vi "log analysis_gps.vi"() -> ()   [LabVIEW 2019] (continued)
0.4317,0.3028,0.5934,0.1135,0.0949,0.0816,0.0957,0.0998,5.2642,0f000001,0*80882a82\n\t", "INSPVAXA,USB3,0,48.5,FINESTEERING,2107,283990.000,02000000,471d,15824;INS_ALIGNMENT_COMPLETE,INS_RTKFIXED,37.37029204407,126.72099699457,9.6988,22.3000,-0.3771,-0.2894,0.0402,-1.247584491,0.667932801,212.987583360,0.4317,0.3028,0.5934,0.1135,0.0949,0.0816,0.0957,0.0998,5.2642,0f000001,0*cfed9a10\n\t", "INSPVAXA,USB3,0,50.0,FINESTEERING,2107,283990.500,02000000,471d,15824;INS_ALIGNMENT_COMPLETE,INS_RTKFIXED,37.37029029580,126.72099542809,9.7025,22.3000,-0.3670,-0.2925,0.0054,-1.144620935,0.833749283,212.845661627,0.4315,0.3031,0.5931,0.1131,0.0946,0.0813,0.0957,0.0998,5.2654,0f000001,0*19c2a41b\n\t", "INSPVAXA,USB3,0,50.0,FINESTEERING,2107,283991.000,02000000,471d,15824;INS_ALIGNMENT_COMPLETE,INS_RTKFIXED,37.37028854245,126.72099383471,9.7082,22.3000,-0.3734,-0.2981,0.0505,-1.053794581,0.860705414,212.916628462,0.4315,0.3031,0.5931,0.1131,0.0946,0.0813,0.0957,0.0998,5.2654,0f000001,0*6cd9c21a\n\t", "INSPVAXA,USB3,0,50.0,FINESTEERING,2107,283991.500,02000000,471d,15824;INS_ALIGNMENT_COMPLETE,INS_RTKFIXED,37.37028678118,126.72099223881,9.7128,22.3000,-0.3905,-0.2870,0.0338,-1.308863276,0.828346639,212.947096436,0.4317,0.3031,0.5932,0.1128,0.0940,0.0810,0.0956,0.0998,5.2662,0f000001,0*9682182f\n\t", "INSPVAXA,USB3,0,50.0,FINESTEERING,2107,283992.000,02000000,471d,15824;INS_ALIGNMENT_COMPLETE,INS_RTKFIXED,37.37028506885,126.72099063831,9.7202,22.3000,-0.3587,-0.3008,0.0194,-1.224018986,0.834141555,212.863695719,0.4317,0.3031,0.5932,0.1128,0.0940,0.0810,0.0956,0.0998,5.2662,0f000001,0*43bde827\n\t", "INSPVAXA,USB3,0,45.0,FINESTEERING,2107,283992.500,02000000,471d,15824;INS_ALIGNMENT_COMPLETE,INS_RTKFIXED,37.37028333459,126.72098904452,9.7257,22.3000,-0.3784,-0.2965,0.0443,-1.050562507,0.745679158,212.979675556,0.4319,0.3033,0.5933,0.1130,0.0942,0.0816,0.0956,0.0997,5.2672,0f000001,0*f6d38c7c\n\t", "INSPVAXA,USB3,0,45.0,FINESTEERING,2107,283993.000,02000000,471d,15824;INS_ALIGNMENT_COMPLETE,INS_RTKFIXED,37.37028161694,126.72098748507,9.7305,22.3000,-0.3588,-0.2835,0.0413,-1.341951739,0.883295300,213.030480888,0.4319,0.3033,0.5933,0.1130,0.0942,0.0816,0.0956,0.0997,5.2672,0f000001,0*8bfaad14\n\t", "INSPVAXA,USB3,0,49.0,FINESTEERING,2107,283993.500,02000000,471d,15824;INS_ALIGNMENT_COMPLETE,INS_RTKFIXED,37.37027987729,126.72098589860,9.7339,22.3000,-0.3886,-0.3118,0.0118,-1.186705860,0.635599144,213.040521206,0.4318,0.3035,0.5934,0.1127,0.0938,0.0813,0.0956,0.0997,5.2685,0f000001,0*5b9abbf8\n\t", "INSPVAXA,USB3,0,49.0,FINESTEERING,2107,283994.000,02000000,471d,15824;INS_ALIGNMENT_COMPLETE,INS_RTKFIXED,37.37027813856,126.72098430051,9.7386,22.3000,-0.3794,-0.2983,0.0413,-1.126640911,0.427805755,213.093758144,0.4318,0.3035,0.5934,0.1127,0.0938,0.0813,0.0956,0.0997,5.2685,0f000001,0*e42dd86e\n\t", "INSPVAXA,USB3,0,41.5,FINESTEERING,2107,283994.500,02000000,471d,15824;INS_ALIGNMENT_COMPLETE,INS_RTKFIXED,37.37027639241,126.72098271837,9.7433,22.3000,-0.3724,-0.2941,0.0395,-1.023992417,0.392331965,213.143460080,0.4318,0.3036,0.5935,0.1130,0.0944,0.0820,0.0956,0.0997,5.2698,0f000001,0*0337d50d\n\t", "INSPVAXA,USB3,0,41.5,FINESTEERING,2107,283995.000,02000000,471d,15824;INS_ALIGNMENT_COMPLETE,INS_RTKFIXED,37.37027465637,126.72098113948,9.7472,22.3000,-0.3708,-0.2998,0.0087,-1.064940932,0.419900141,213.213279076,0.4318,0.3036,0.5935,0.1130,0.0944,0.0820,0.0956,0.0997,5.2698,0f000001,0*335ddb23\n\t", "INSPVAXA,USB3,0,49.5,FINESTEERING,2107,283995.500,02000000,471d,15824;INS_ALIGNMENT_COMPLETE,INS_RTKFIXED,37.37027293232,126.72097957470,9.7494,22.3000,-0.3727,-0.2928,0.0273,-1.114629129,0.419021826,213.334562050,0.4319,0.3032,0.5939,0.1127,0.0939,0.0817,0.0957,0.0997,5.2708,0f000001,0*bec96f91\n\t", "INSPVAXA,USB3,0,49.5,FINESTEERING,2107,283996.000,02000000,471d,15824;INS_ALIGNMENT_COMPLETE,INS_RTKFIXED,37.37027121924,126.72097799640,9.7538,22.3000,-0.3785,-0.2972,0.0344,-0.912805448,0.531088142,213.375963340,0.4319,0.3032,0.5939,0.1127,0.0939,0.0817,0.0957,0.0997,5.2708,0f000001,0*e0fc992c\n\t", "INSPVAXA,USB3,0,48.5,FINESTEERING,2107,283996.500,02000000,471d,15824;INS_ALIGNMENT_COMPLETE,INS_RTKFIXED,37.37026950707,126.72097642523,9.7575,22.3000,-0.3790,-0.2971,0.0045,-1.031000712,0.442701672,213.487798192,0.4317,0.3031,0.5940,0.1124,0.0936,0.0813,0.0957,0.0997,5.2719,0f000001,0*6ebbd163\n\t", "INSPVAXA,USB3,0,48.5,FINESTEERING,2107,283997.000,02000000,471d,15824;INS_ALIGNMENT_COMPLETE,INS_RTKFIXED,37.37026778904,126.72097482944,9.7613,22.3000,-0.3776,-0.3087,0.0370,-1.077110117,0.533414002,213.644467670,0.4317,0.3031,0.5940,0.1124,0.0936,0.0813,0.0957,0.0997,5.2719,0f000001,0*eda6f981\n\t", "INSPVAXA,USB3,0,51.5,FINESTEERING,2107,283997.500,02000000,471d,15824;INS_ALIGNMENT_COMPLETE,INS_RTKFIXED,37.37026610502,126.72097322741,9.7652,22.3000,-0.3735,-0.2926,0.0418,-0.879042002,0.635388403,213.712940335,0.4318,0.3033,0.5943,0.1122,0.0934,0.0810,0.0958,0.0998,5.2733,0f000001,0*c5914784\n\t", "INSPVAXA,USB3,0,51.5,FINESTEERING,2107,283998.000,02000000,471d,15824;INS_ALIGNMENT_COMPLETE,INS_RTKFIXED,37.37026439172,126.72097159305,9.7705,22.3000,-0.3793,-0.3043,0.0231,-0.804340415,0.481108177,213.810502820,0.4318,0.3033,0.5943,0.1122,0.0934,0.0810,0.0958,0.0998,5.2733,0f000001,0*97086bfc\n\t", "INSPVAXA,USB3,0,51.0,FINESTEERING,2107,283998.500,02000000,471d,15824;INS_ALIGNMENT_COMPLETE,INS_RTKFIXED,37.37026268780,126.72097001383,9.7729,22.3000,-0.3715,-0.3065,0.0247,-0.969252583,0.581649669,213.913706075,0.4317,0.3034,0.5943,0.1125,0.0938,0.0813,0.0958,0.0998,5.2748,0f000001,0*e268e54b\n\t", "INSPVAXA,USB3,0,51.0,FINESTEERING,2107,283999.000,02000000,471d,15824;INS_ALIGNMENT_COMPLETE,INS_RTKFIXED,37.37026095503,126.72096836486,9.7766,22.3000,-0.3661,-0.3031,0.0412,-0.630265217,0.537624421,214.046710084,0.4317,0.3034,0.5943,0.1125,0.0938,0.0813,0.0958,0.0998,5.2748,0f000001,0*95a9afe3\n\t", "INSPVAXA,USB3,0,49.5,FINESTEERING,2107,283999.500,02000000,471d,15824;INS_ALIGNMENT_COMPLETE,INS_RTKFIXED,37.37025925101,126.72096675133,9.7788,22.3000,-0.3833,-0.2925,0.0276,-0.676998170,0.665326171,214.262149706,0.4315,0.3034,0.5944,0.1124,0.0937,0.0810,0.0958,0.0998,5.2762,0f000001,0*6af82f9f\n\t", "DUALANTENNAHEADINGA,USB3,0,49.5,FINESTEERING,2107,284000.000,02000000,d426,15824;INSUFFICIENT_OBS,NONE,-1.000000000,0.000000000,0.000000000,0.0,0.000000000,0.000000000,\"631T\",10,3,3,3,04,00,20,00*77bc98b4\n\t", "INSPVAXA,USB3,0,51.5,FINESTEERING,2107,284000.500,02000000,471d,15824;INS_ALIGNMENT_COMPLETE,INS_RTKFIXED,37.37025584789,126.72096350983,9.7893,22.3000,-0.3628,-0.2938,0.0413,-0.857969709,0.678060682,214.382554495,0.4312,0.3037,0.5943,0.1122,0.0935,0.0807,0.0958,0.0998,5.2776,0f000001,0*ebd8e3c0\n\t", "INSPVAXA,USB3,0,51.5,FINESTEERING,2107,284001.000,02000000,471d,15824;INS_ALIGNMENT_COMPLETE,INS_RTKFIXED,37.37025415125,126.72096186926,9.7945,22.3000,-0.3741,-0.3078,0.0321,-0.868538574,0.838914865,214.492970647,0.4312,0.3037,0.5943,0.1122,0.0935,0.0807,0.0958,0.0998,5.2776,0f000001,0*3e03e893\n\t", "INSPVAXA,USB3,0,51.5,FINESTEERING,2107,284001.500,02000000,471d,15824;INS_ALIGNMENT_COMPLETE,INS_RTKFIXED,37.37025245958,126.72096024152,9.7991,22.3000,-0.3759,-0.3085,0.0182,-0.727729305,0.679989814,214.645667926,0.4313,0.3035,0.5942,0.1121,0.0935,0.0804,0.0958,0.0999,5.2791,0f000001,0*dc1168a6\n\t", "INSPVAXA,USB3,0,51.5,FINESTEERING,2107,284002.000,02000000,471d,15824;INS_ALIGNMENT_COMPLETE,INS_RTKFIXED,37.37025076480,126.72095861170,9.8045,22.3000,-0.3744,-0.3095,0.0470,-0.816843186,0.787318201,214.620444446,0.4313,0.3035,0.5942,0.1121,0.0935,0.0804,0.0958,0.0999,5.2791,0f000001,0*a2e8b743\n\t", "INSPVAXA,USB3,0,51.5,FINESTEERING,2107,284002.500,02000000,471d,15824;INS_ALIGNMENT_COMPLETE,INS_RTKFIXED,37.37024907128,126.72095697824,9.8087,22.3000,-0.3691,-0.2994,0.0299,-0.885724025,0.937533929,214.679042241,0.4311,0.3036,0.5939,0.1121,0.0934,0.0802,0.0958,0.0999,5.2806,0f000001,0*c448775c\n\t", "INSPVAXA,USB3,0,51.5,FINESTEERING,2107,284003.000,02000000,471d,15824;INS_ALIGNMENT_COMPLETE,INS_RTKFIXED,37.37024737149,126.72095529976,9.8122,22.3000,-0.3776,-0.3159,0.0244,-0.547028991,0.805451972,214.632048591,0.4311,0.3036,0.5939,0.1121,0.0934,0.0802,0.0958,0.0999,5.2806,0f000001,0*63822f21\n\t", "INSPVAXA,USB3,0,51.5,FINESTEERING,2107,284003.500,02000000,471d,15824;INS_ALIGNMENT_COMPLETE,INS_RTKFIXED,37.37024569352,126.72095368049,9.8164,22.3000,-0.3735,-0.3059,0.0298,-0.766116345,0.775309427,214.637421132,0.4311,0.3038,0.5936,0.1120,0.0934,0.0800,0.0957,0.0999,5.2822,0f000001,0*13581e5f\n\t", "INSPVAXA,USB3,0,51.5,FINESTEERING,2107,284004.000,02000000,471d,15824;INS_ALIGNMENT_COMPLETE,INS_RTKFIXED,37.37024397579,126.72095202035,9.8197,22.3000,-0.3785,-0.3116,0.0275,-0.938815319,0.810465745,214.701472535,0.4311,0.3038,0.5936,0.1120,0.0934,0.0800,0.0957,0.0999,5.2822,0f000001,0*789baddb\n\t", "DUALANTENNAHEADINGA,USB3,0,47.5,FINESTEERING,2107,284004.500,02000000,d426,15824;INSUFFICIENT_OBS,NONE,-1.000000000,0.000000000,0.000000000,0.0,0.000000000,0.000000000,\"631T\",10,3,3,3,04,00,20,00*da91d4f3\n\t", "INSPVAXA,USB3,0,47.5,FINESTEERING,2107,284005.000,02000000,471d,15824;INS_ALIGNMENT_COMPLETE,INS_RTKFIXED,37.37024061401,126.72094879160,9.8273,22.3000,-0.3519,-0.2880,0.0226,-1.106323237,0.920552674,214.656768250,0.4310,0.3041,0.5933,0.1128,0.0943,0.0811,0.0957,0.0998,5.2837,0f000001,0*6ae8f33a\n\t", "DUALANTENNAHEADINGA,USB3,0,51.5,FINESTEERING,2107,284005.500,02000000,d426,15824;INSUFFICIENT_OBS,NONE,-1.000000000,0.000000000,0.000000000,0.0,0.000000000,0.000000000,\"631T\",10,3,3,3,04,00,20,00*e47d0294\n\t", "DUALANTENNAHEADINGA,USB3,0,51.5,FINESTEERING,2107,284006.000,02000000,d426,15824;INSUFFICIENT_OBS,NONE,-1.000000000,0.000000000,0.000000000,0.0,0.000000000,0.000000000,\"631T\",11,3,3,3,04,00,20,00*52e49efe\n\t", "INSPVAXA,USB3,0,53.0,FINESTEERING,2107,284006.500,02000000,471d,15824;INS_ALIGNMENT_COMPLETE,INS_RTKFIXED,37.37023555537,126.72094390060,9.8375,22.3000,-0.3979,-0.3155,0.0300,-1.049604395,0.780641756,214.313549456,0.4317,0.3045,0.5932,0.1125,0.0938,0.0806,0.0956,0.0998,5.2867,0f000001,0*baf56160\n\t", "DUALANTENNAHEADINGA,USB3,0,53.0,FINESTEERING,2107,284007.000,02000000,d426,15824;INSUFFICIENT_OBS,NONE,-1.000000000,0.000000000,0.000000000,0.0,0.000000000,0.000000000,\"631T\",11,3,3,3,04,00,20,00*a2cfd1a3\n\t", "INSPVAXA,USB3,0,51.5,FINESTEERING,2107,284007.500,02000000,471d,15824;INS_ALIGNMENT_COMPLETE,INS_RTKFIXED,37.37023216601,126.72094065037,9.8419,22.3000,-0.3656,-0.2859,0.0240,-0.929585052,0.783187506,214.018400547,0.4319,0.3042,0.5932,0.1130,0.0943,0.0814,0.0956,0.0998,5.2881,0f000001,0*b155cbfb\n\t", "INSPVAXA,USB3,0,51.5,FINESTEERING,2107,284008.000,02000000,471d,15824;INS_ALIGNMENT_COMPLETE,INS_RTKFIXED,37.37023049066,126.72093905511,9.8436,22.3000,-0.3675,-0.2972,0.0326,-1.081497544,1.069523498,213.947516981,0.4319,0.3042,0.5932,0.1130,0.0943,0.0814,0.0956,0.0998,5.2881,0f000001,0*b15b7ce2\n\t", "DUALANTENNAHEADINGA,USB3,0,50.5,FINESTEERING,2107,284008.500,02000000,d426,15824;INSUFFICIENT_OBS,NONE,-1.000000000,0.000000000,0.000000000,0.0,0.000000000,0.000000000,\"631T\",10,3,3,3,04,00,20,00*59d2ef86\n\t", "INSPVAXA,USB3,0,50.5,FINESTEERING,2107,284009.000,02000000,471d,15824;INS_ALIGNMENT_COMPLETE,INS_RTKFIXED,37.37022706155,126.72093581324,9.8448,22.3000,-0.3775,-0.3022,0.0342,-1.257860345,0.478173626,213.753744794,0.4320,0.3040,0.5934,0.1130,0.0939,0.0812,0.0956,0.0998,5.2894,0f000001,0*088bd23f\n\t", "DUALANTENNAHEADINGA,USB3,0,50.0,FINESTEERING,2107,284009.500,02000000,d426,15824;INSUFFICIENT_OBS,NONE,-1.000000000,0.000000000,0.000000000,0.0,0.000000000,0.000000000,\"631T\",12,3,3,3,04,00,20,00*15c40b62\n\t", "DUALANTENNAHEADINGA,USB3,0,50.0,FINESTEERING,2107,284010.000,02000000,d426,15824;INSUFFICIENT_OBS,NONE,-1.000000000,0.000000000,0.000000000,0.0,0.000000000,0.000000000,\"631T\",11,3,3,3,04,00,20,00*2b190075\n\t", "DUALANTENNAHEADINGA,USB3,0,52.0,FINESTEERING,2107,284010.500,02000000,d426,15824;INSUFFICIENT_OBS,NONE,-1.000000000,0.000000000,0.000000000,0.0,0.000000000,0.000000000,\"631T\",11,3,3,3,04,00,20,00*3483bc64\n\t", "DUALANTENNAHEADINGA,USB3,0,52.0,FINESTEERING,2107,284011.000,02000000,d426,15824;INSUFFICIENT_OBS,NONE,-1.000000000,0.000000000,0.000000000,0.0,0.000000000,0.000000000,\"631T\",10,3,3,3,04,00,20,00*59aa29bc\n\t", "DUALANTENNAHEADINGA,USB3,0,50.0,FINESTEERING,2107,284011.500,02000000,d426,15824;INSUFFICIENT_OBS,NONE,-1.000000000,0.000000000,0.000000000,0.0,0.000000000,0.000000000,\"631T\",10,3,3,3,04,00,20,00*463095ad\n\t", "DUALANTENNAHEADINGA,USB3,0,50.0,FINESTEERING,2107,284012.000,02000000,d426,15824;INSUFFICIENT_OBS,NONE,-1.000000000,0.000000000,0.000000000,0.0,0.000000000,0.000000000,\"631T\",11,3,3,3,04,00,20,00*f0a909c7\n\t", "INSPVAXA,USB3,0,52.0,FINESTEERING,2107,284012.500,02000000,471d,15824;INS_ALIGNMENT_COMPLETE,INS_RTKFIXED,37.37021521893,126.72092466142,9.8618,22.3000,-0.3847,-0.3021,0.0234,-0.775837810,0.832251652,213.741589159,0.4316,0.3037,0.5939,0.1121,0.0935,0.0807,0.0957,0.0997,5.2927,0f000001,0*15662a94\n\t", "DUALANTENNAHEADINGA,USB3,0,52.0,FINESTEERING,2107,284013.000,02000000,d426,15824;INSUFFICIENT_OBS,NONE,-1.000000000,0.000000000,0.000000000,0.0,0.000000000,0.000000000,\"631T\",11,3,3,3,04,00,20,00*55f8a056\n\t", "DUALANTENNAHEADINGA,USB3,0,49.0,FINESTEERING,2107,284013.500,02000000,d426,15824;INSUFFICIENT_OBS,NONE,-1.000000000,0.000000000,0.000000000,0.0,0.000000000,0.000000000,\"631T\",10,3,3,3,04,00,20,00*bcdfd03e\n\t", "DUALANTENNAHEADINGA,USB3,0,49.0,FINESTEERING,2107,284014.000,02000000,d426,15824;INSUFFICIENT_OBS,NONE,-1.000000000,0.000000000,0.000000000,0.0,0.000000000,0.000000000,\"631T\",10,3,3,3,04,00,20,00*b1b5d929\n\t", "DUALANTENNAHEADINGA,USB3,0,48.0,FINESTEERING,2107,284014.500,02000000,d426,15824;INSUFFICIENT_OBS,NONE,-1.000000000,0.000000000,0.000000000,0.0,0.000000000,0.000000000,\"631T\",11,3,3,3,04,00,20,00*d5009e8c\n\t", "INSPVAXA,USB3,0,48.0,FINESTEERING,2107,284015.000,02000000,471d,15824;INS_ALIGNMENT_COMPLETE,INS_RTKFIXED,37.37020683430,126.72091660839,9.8841,22.3000,-0.3478,-0.2798,0.0325,-1.211016237,0.525489122,214.520046866,0.4313,0.3041,0.5940,0.1119,0.0933,0.0802,0.0957,0.0997,5.2955,0f000001,0*ac9f229d\n\t", "INSPVAXA,USB3,0,50.5,FINESTEERING,2107,284015.500,02000000,471d,15824;INS_ALIGNMENT_COMPLETE,INS_RTKFIXED,37.37020518291,126.72091499411,9.8875,22.3000,-0.3472,-0.2997,0.0277,-1.071436018,0.954919930,214.713975272,0.4312,0.3037,0.5941,0.1119,0.0933,0.0800,0.0957,0.0997,5.2971,0f000001,0*82bfde41\n\t", "INSPVAXA,USB3,0,50.5,FINESTEERING,2107,284016.000,02000000,471d,15824;INS_ALIGNMENT_COMPLETE,INS_RTKFIXED,37.37020352454,126.72091333889,9.8896,22.3000,-0.3642,-0.3113,0.0147,-0.944083303,0.844230452,215.071518379,0.4312,0.3037,0.5941,0.1119,0.0933,0.0800,0.0957,0.0997,5.2971,0f000001,0*acd4ef81\n\t", "DUALANTENNAHEADINGA,USB3,0,48.0,FINESTEERING,2107,284016.500,02000000,d426,15824;INSUFFICIENT_OBS,NONE,-1.000000000,0.000000000,0.000000000,0.0,0.000000000,0.000000000,\"631T\",11,3,3,3,04,00,20,00*0eb0973e\n\t", "DUALANTENNAHEADINGA,USB3,0,48.0,FINESTEERING,2107,284017.000,02000000,d426,15824;INSUFFICIENT_OBS,NONE,-1.000000000,0.000000000,0.000000000,0.0,0.000000000,0.000000000,\"631T\",10,3,3,3,04,00,20,00*639902e6\n\t", "DUALANTENNAHEADINGA,USB3,0,46.5,FINESTEERING,2107,284017.500,02000000,d426,15824;INSUFFICIENT_OBS,NONE,-1.000000000,0.000000000,0.000000000,0.0,0.000000000,0.000000000,\"631T\",10,3,3,3,04,00,20,00*f7dfbd48\n\t", "DUALANTENNAHEADINGA,USB3,0,46.5,FINESTEERING,2107,284018.000,02000000,d426,15824;INSUFFICIENT_OBS,NONE,-1.000000000,0.000000000,0.000000000,0.0,0.000000000,0.000000000,\"631T\",10,3,3,3,04,00,20,00*22979e15\n\t", "DUALANTENNAHEADINGA,USB3,0,48.0,FINESTEERING,2107,284018.500,02000000,d426,15824;INSUFFICIENT_OBS,NONE,-1.000000000,0.000000000,0.000000000,0.0,0.000000000,0.000000000,\"631T\",11,3,3,3,04,00,20,00*6133a1e3\n\t", "DUALANTENNAHEADINGA,USB3,0,48.0,FINESTEERING,2107,284019.000,02000000,d426,15824;INSUFFICIENT_OBS,NONE,-1.000000000,0.000000000,0.000000000,0.0,0.000000000,0.000000000,\"631T\",13,3,3,3,04,00,20,00*af4cb292\n\t", "DUALANTENNAHEADINGA,USB3,0,50.0,FINESTEERING,2107,284019.500,02000000,d426,15824;INSUFFICIENT_OBS,NONE,-1.000000000,0.000000000,0.000000000,0.0,0.000000000,0.000000000,\"631T\",12,3,3,3,04,00,20,00*eaa6b916\n\t", "DUALANTENNAHEADINGA,USB3,0,50.0,FINESTEERING,2107,284020.000,02000000,d426,15824;INSUFFICIENT_OBS,NONE,-1.000000000,0.000000000,0.000000000,0.0,0.000000000,0.000000000,\"631T\",10,3,3,3,04,00,20,00*262d50f0\n\t", "DUALANTENNAHEADINGA,USB3,0,48.5,FINESTEERING,2107,284020.500,02000000,d426,15824;INSUFFICIENT_OBS,NONE,-1.000000000,0.000000000,0.000000000,0.0,0.000000000,0.000000000,\"631T\",9,3,3,3,04,00,20,00*7dfaf070\n\t", "DUALANTENNAHEADINGA,USB3,0,48.5,FINESTEERING,2107,284021.000,02000000,d426,15824;INSUFFICIENT_OBS,NONE,-1.000000000,0.000000000,0.000000000,0.0,0.000000000,0.000000000,\"631T\",9,3,3,3,04,00,20,00*66d97584\n\t", "DUALANTENNAHEADINGA,USB3,0,51.5,FINESTEERING,2107,284021.500,02000000,d426,15824;INSUFFICIENT_OBS,NONE,-1.000000000,0.000000000,0.000000000,0.0,0.000000000,0.000000000,\"631T\",10,3,3,3,04,00,20,00*add87518\n\t", "DUALANTENNAHEADINGA,USB3,0,51.5,FINESTEERING,2107,284022.000,02000000,d426,15824;INSUFFICIENT_OBS,NONE,-1.000000000,0.000000000,0.000000000,0.0,0.000000000,0.000000000,\"631T\",11,3,3,3,04,00,20,00*1b41e972\n\t", "DUALANTENNAHEADINGA,USB3,0,51.0,FINESTEERING,2107,284022.500,02000000,d426,15824;INSUFFICIENT_OBS,NONE,-1.000000000,0.000000000,0.000000000,0.0,0.000000000,0.000000000,\"631T\",11,3,3,3,04,00,20,00*99281ee7\n\t", "DUALANTENNAHEADINGA,USB3,0,51.0,FINESTEERING,2107,284023.000,02000000,d426,15824;INSUFFICIENT_OBS,NONE,-1.000000000,0.000000000,0.000000000,0.0,0.000000000,0.000000000,\"631T\",11,3,3,3,04,00,20,00*23e30b67\n\t", "DUALANTENNAHEADINGA,USB3,0,48.5,FINESTEERING,2107,284023.500,02000000,d426,15824;INSUFFICIENT_OBS,NONE,-1.000000000,0.000000000,0.000000000,0.0,0.000000000,0.000000000,\"631T\",11,3,3,3,04,00,20,00*80d5b0d3\n\t", "DUALANTENNAHEADINGA,USB3,0,50.5,FINESTEERING,2107,284025.000,02000000,d426,15824;INSUFFICIENT_OBS,NONE,-1.000000000,0.000000000,0.000000000,0.0,0.000000000,0.000000000,\"631T\",12,3,3,3,04,00,20,00*062aa131\n\t", "DUALANTENNAHEADINGA,USB3,0,50.0,FINESTEERING,2107,284025.500,02000000,d426,15824;INSUFFICIENT_OBS,NONE,-1.000000000,0.000000000,0.000000000,0.0,0.000000000,0.000000000,\"631T\",11,3,3,3,04,00,20,00*2715d00d\n\t", "DUALANTENNAHEADINGA,USB3,0,50.0,FINESTEERING,2107,284026.000,02000000,d426,15824;INSUFFICIENT_OBS,NONE,-1.000000000,0.000000000,0.000000000,0.0,0.000000000,0.000000000,\"631T\",11,3,3,3,04,00,20,00*466ecc3f\n\t", "DUALANTENNAHEADINGA,USB3,0,52.0,FINESTEERING,2107,284026.500,02000000,d426,15824;INSUFFICIENT_OBS,NONE,-1.000000000,0.000000000,0.000000000,0.0,0.000000000,0.000000000,\"631T\",11,3,3,3,04,00,20,00*59f4702e\n\t", "DUALANTENNAHEADINGA,USB3,0,52.0,FINESTEERING,2107,284027.000,02000000,d426,15824;INSUFFICIENT_OBS,NONE,-1.000000000,0.000000000,0.000000000,0.0,0.000000000,0.000000000,\"631T\",11,3,3,3,04,00,20,00*e33f65ae\n\t", "DUALANTENNAHEADINGA,USB3,0,51.0,FINESTEERING,2107,284027.500,02000000,d426,15824;INSUFFICIENT_OBS,NONE,-1.000000000,0.000000000,0.000000000,0.0,0.000000000,0.000000000,\"631T\",11,3,3,3,04,00,20,00*98e10f1b\n\t", "DUALANTENNAHEADINGA,USB3,0,51.0,FINESTEERING,2107,284028.000,02000000,d426,15824;INSUFFICIENT_OBS,NONE,-1.000000000,0.000000000,0.000000000,0.0,0.000000000,0.000000000,\"631T\",12,3,3,3,04,00,20,00*eeffaaef\n\t", "INSPVAXA,USB3,0,53.0,FINESTEERING,2107,284028.500,02000000,471d,15824;INS_ALIGNMENT_COMPLETE,INS_RTKFIXED,37.37016418129,126.72086876057,9.9277,22.3000,-0.3056,-0.3533,0.0249,-0.407357683,-0.326305353,221.094375999,0.4345,0.3056,0.5971,0.1128,0.0942,0.0822,0.0958,0.1003,5.3097,0f000001,0*9e144474\n\t", "DUALANTENNAHEADINGA,USB3,0,53.0,FINESTEERING,2107,284029.000,02000000,d426,15824;INSUFFICIENT_OBS,NONE,-1.000000000,0.000000000,0.000000000,0.0,0.000000000,0.000000000,\"631T\",11,3,3,3,04,00,20,00*e8f885d7\n\t", "DUALANTENNAHEADINGA,USB3,0,48.5,FINESTEERING,2107,284029.500,02000000,d426,15824;INSUFFICIENT_OBS,NONE,-1.000000000,0.000000000,0.000000000,0.0,0.000000000,0.000000000,\"631T\",11,3,3,3,04,00,20,00*8347932b\n\t", "DUALANTENNAHEADINGA,USB3,0,48.5,FINESTEERING,2107,284030.000,02000000,d426,15824;INSUFFICIENT_OBS,NONE,-1.000000000,0.000000000,0.000000000,0.0,0.000000000,0.000000000,\"631T\",13,3,3,3,04,00,20,00*6a781864\n\t", "DUALANTENNAHEADINGA,USB3,0,50.0,FINESTEERING,2107,284030.500,02000000,d426,15824;INSUFFICIENT_OBS,NONE,-1.000000000,0.000000000,0.000000000,0.0,0.000000000,0.000000000,\"631T\",15,3,3,3,04,00,20,00*30d67e67\n\t", "DUALANTENNAHEADINGA,USB3,0,50.0,FINESTEERING,2107,284031.000,02000000,d426,15824;INSUFFICIENT_OBS,NONE,-1.000000000,0.000000000,0.000000000,0.0,0.000000000,0.000000000,\"631T\",14,3,3,3,04,00,20,00*5dffebbf\n\t", "DUALANTENNAHEADINGA,USB3,0,46.0,FINESTEERING,2107,284031.500,02000000,d426,15824;INSUFFICIENT_OBS,NONE,-1.000000000,0.000000000,0.000000000,0.0,0.000000000,0.000000000,\"631T\",14,3,3,3,04,00,20,00*d9d82858\n\t", "DUALANTENNAHEADINGA,USB3,0,46.0,FINESTEERING,2107,284032.000,02000000,d426,15824;INSUFFICIENT_OBS,NONE,-1.000000000,0.000000000,0.000000000,0.0,0.000000000,0.000000000,\"631T\",15,3,3,3,04,00,20,00*6f41b432\n\t", "INSPVAXA,USB3,0,49.0,FINESTEERING,2107,284032.550,02000000,471d,15824;INS_ALIGNMENT_COMPLETE,INS_RTKFIXED,37.37015203193,126.72085320398,9.9212,22.3000,-0.2929,-0.3693,0.0073,-0.969546435,-0.769890504,222.991083315,0.4327,0.3047,0.5976,0.1132,0.0946,0.0822,0.0960,0.1005,5.3138,0f000001,0*7ab4b638\n\t", "INSPVAXA,USB3,0,49.0,FINESTEERING,2107,284033.050,02000000,471d,15824;INS_ALIGNMENT_COMPLETE,INS_RTKFIXED,37.37015056233,126.72085129060,9.9204,22.3000,-0.2846,-0.3575,0.0263,-1.291425678,-0.544067497,223.276181185,0.4326,0.3039,0.5975,0.1132,0.0942,0.0818,0.0959,0.1005,5.3153,0f000001,0*1faf9100\n\t", "INSPVAXA,USB3,0,49.5,FINESTEERING,2107,284033.550,02000000,471d,15824;INS_ALIGNMENT_COMPLETE,INS_RTKFIXED,37.37014911453,126.72084937010,9.9197,22.3000,-0.2886,-0.3722,0.0073,-1.220668676,-0.203530913,223.385400784,0.4326,0.3039,0.5975,0.1132,0.0942,0.0818,0.0959,0.1005,5.3153,0f000001,0*08db545a\n\t", "DUALANTENNAHEADINGA,USB3,0,53.5,FINESTEERING,2107,284034.500,02000000,d426,15824;INSUFFICIENT_OBS,NONE,-1.000000000,0.000000000,0.000000000,0.0,0.000000000,0.000000000,\"631T\",13,3,3,3,04,00,20,00*38acfd71\n\t", "DUALANTENNAHEADINGA,USB3,0,53.5,FINESTEERING,2107,284035.000,02000000,d426,15824;INSUFFICIENT_OBS,NONE,-1.000000000,0.000000000,0.000000000,0.0,0.000000000,0.000000000,\"631T\",13,3,3,3,04,00,20,00*8267e8f1\n\t", "DUALANTENNAHEADINGA,USB3,0,48.5,FINESTEERING,2107,284035.500,02000000,d426,15824;INSUFFICIENT_OBS,NONE,-1.000000000,0.000000000,0.000000000,0.0,0.000000000,0.000000000,\"631T\",12,3,3,3,04,00,20,00*6b409899\n\t", "INSPVAXA,USB3,0,48.5,FINESTEERING,2107,284036.050,02000000,471d,15824;INS_ALIGNMENT_COMPLETE,INS_RTKFIXED,37.37014185776,126.72083957018,9.9201,22.3000,-0.2874,-0.3754,0.0180,-1.581713384,-0.281316451,224.309302807,0.4333,0.3030,0.5980,0.1134,0.0944,0.0817,0.0958,0.1004,5.3150,0f000001,0*fb9a3949\n\t", "DUALANTENNAHEADINGA,USB3,0,49.0,FINESTEERING,2107,284037.000,02000000,d426,15824;INSUFFICIENT_OBS,NONE,-1.000000000,0.000000000,0.000000000,0.0,0.000000000,0.000000000,\"631T\",12,3,3,3,04,00,20,00*56ddb01a\n\t", "DUALANTENNAHEADINGA,USB3,0,50.5,FINESTEERING,2107,284038.000,02000000,d426,15824;INSUFFICIENT_OBS,NONE,-1.000000000,0.000000000,0.000000000,0.0,0.000000000,0.000000000,\"631T\",12,3,3,3,04,00,20,00*20a328f3\n\t", "INSPVAXA,USB3,0,49.0,FINESTEERING,2107,284038.550,02000000,471d,15824;INS_ALIGNMENT_COMPLETE,INS_RTKFIXED,37.37013464151,126.72082964109,9.9222,22.3000,-0.2992,-0.3861,0.0057,-1.451445202,0.305563653,224.751611567,0.4334,0.3031,0.5974,0.1129,0.0939,0.0810,0.0957,0.1002,5.3127,0f000001,0*124febdb\n\t", "DUALANTENNAHEADINGA,USB3,0,49.0,FINESTEERING,2107,284039.000,02000000,d426,15824;INSUFFICIENT_OBS,NONE,-1.000000000,0.000000000,0.000000000,0.0,0.000000000,0.000000000,\"631T\",12,3,3,3,04,00,20,00*395e86c7\n\t", "INSPVAXA,USB3,0,52.5,FINESTEERING,2107,284039.550,02000000,471d,15824;INS_ALIGNMENT_COMPLETE,INS_RTKFIXED,37.37013171453,126.72082571208,9.9282,22.3000,-0.2895,-0.3679,0.0213,-1.368726775,0.328135846,224.170943357,0.4333,0.3035,0.5969,0.1130,0.0937,0.0807,0.0957,0.1001,5.3122,0f000001,0*6a698e8e\n\t", "DUALANTENNAHEADINGA,USB3,0,52.5,FINESTEERING,2107,284040.000,02000000,d426,15824;INSUFFICIENT_OBS,NONE,-1.000000000,0.000000000,0.000000000,0.0,0.000000000,0.000000000,\"631T\",12,3,3,3,04,00,20,00*a1b6ba7e\n\t", "DUALANTENNAHEADINGA,USB3,0,51.5,FINESTEERING,2107,284040.500,02000000,d426,15824;INSUFFICIENT_OBS,NONE,-1.000000000,0.000000000,0.000000000,0.0,0.000000000,0.000000000,\"631T\",13,3,3,3,04,00,20,00*0d8a5093\n\t", "INSPVAXA,USB3,0,49.5,FINESTEERING,2107,284041.050,02000000,471d,15824;INS_ALIGNMENT_COMPLETE,INS_RTKFIXED,37.37012716980,126.72082004347,9.9321,22.3000,-0.3311,-0.3541,0.0307,-1.568797155,-0.218407470,219.720707571,0.4330,0.3038,0.5962,0.1133,0.0947,0.0815,0.0956,0.0999,5.3092,0f000001,0*1a0eaafc\n\t", "DUALANTENNAHEADINGA,USB3,0,49.5,FINESTEERING,2107,284042.000,02000000,d426,15824;INSUFFICIENT_OBS,NONE,-1.000000000,0.000000000,0.000000000,0.0,0.000000000,0.000000000,\"631T\",11,3,3,3,04,00,20,00*3086d40c\n\t", "INSPVAXA,USB3,0,48.5,FINESTEERING,2107,284042.550,02000000,471d,15824;INS_ALIGNMENT_COMPLETE,INS_RTKFIXED,37.37012309586,126.72081639468,9.9287,22.3000,-0.2297,-0.1271,0.0043,-1.454240344,-0.869420112,204.842413707,0.4327,0.3036,0.5960,0.1151,0.0944,0.0812,0.0955,0.0998,5.3038,0f000001,0*d43454d1\n\t", "DUALANTENNAHEADINGA,USB3,0,50.0,FINESTEERING,2107,284044.000,02000000,d426,15824;INSUFFICIENT_OBS,NONE,-1.000000000,0.000000000,0.000000000,0.0,0.000000000,0.000000000,\"631T\",10,3,3,3,04,00,20,00*24e0e22e\n\t", "INSPVAXA,USB3,0,48.5,FINESTEERING,2107,284045.050,02000000,471d,15824;INS_ALIGNMENT_COMPLETE,INS_RTKFIXED,37.37011692256,126.72081439819,9.9167,22.3000,-0.2491,-0.0343,-0.0078,-1.423202522,-1.142665090,179.061069069,0.4321,0.3052,0.5955,0.1145,0.0942,0.0804,0.0954,0.0993,5.2602,0f000001,0*4754f5d4\n\t", "INSPVAXA,USB3,0,52.0,FINESTEERING,2107,284045.550,02000000,471d,15824;INS_ALIGNMENT_COMPLETE,INS_RTKFIXED,37.37011564365,126.72081436501,9.9153,22.3000,-0.2694,0.0262,0.0028,-1.152838671,-0.998441499,173.727062004,0.4321,0.3052,0.5955,0.1145,0.0942,0.0804,0.0954,0.0993,5.2602,0f000001,0*22f8d84c\n\t", "DUALANTENNAHEADINGA,USB3,0,52.0,FINESTEERING,2107,284046.000,02000000,d426,15824;INSUFFICIENT_OBS,NONE,-1.000000000,0.000000000,0.000000000,0.0,0.000000000,0.000000000,\"631T\",11,3,3,3,04,00,20,00*e03bc68c\n\t", "INSPVAXA,USB3,0,51.0,FINESTEERING,2107,284046.550,02000000,471d,15824;INS_ALIGNMENT_COMPLETE,INS_RTKFIXED,37.37011307842,126.72081488040,9.9123,22.3000,-0.2496,0.0473,0.0011,-1.038780714,-0.928259537,163.465097111,0.4314,0.3044,0.5952,0.1141,0.0948,0.0802,0.0953,0.0991,5.2403,0f000001,0*99f045b6\n\t", "INSPVAXA,USB3,0,51.0,FINESTEERING,2107,284047.050,02000000,471d,15824;INS_ALIGNMENT_COMPLETE,INS_RTKFIXED,37.37011184110,126.72081538854,9.9110,22.3000,-0.2193,0.0992,-0.0077,-0.985316738,-1.067024719,158.394367394,0.4310,0.3038,0.5948,0.1149,0.0957,0.0800,0.0951,0.0989,5.2224,0f000001,0*e0578a7c\n\t", "INSPVAXA,USB3,0,51.5,FINESTEERING,2107,284047.550,02000000,471d,15824;INS_ALIGNMENT_COMPLETE,INS_RTKFIXED,37.37011062254,126.72081597469,9.9105,22.3000,-0.2405,0.0932,0.0076,-1.129336312,-1.227184174,152.839130107,0.4310,0.3038,0.5948,0.1149,0.0957,0.0800,0.0951,0.0989,5.2224,0f000001,0*808c7198\n\t", "DUALANTENNAHEADINGA,USB3,0,51.5,FINESTEERING,2107,284048.000,02000000,d426,15824;INSUFFICIENT_OBS,NONE,-1.000000000,0.000000000,0.000000000,0.0,0.000000000,0.000000000,\"631T\",10,3,3,3,04,00,20,00*a1eded29\n\t", "INSPVAXA,USB3,0,51.5,FINESTEERING,2107,284048.550,02008000,471d,15824;INS_ALIGNMENT_COMPLETE,INS_RTKFIXED,37.37010828032,126.72081752863,9.9063,22.3000,-0.2254,0.1193,0.0027,-0.673231023,-1.787802383,142.480422614,0.4310,0.3033,0.5944,0.1159,0.0969,0.0798,0.0949,0.0986,5.2063,0f000001,0*d0854b13\n\t", "INSPVAXA,USB3,0,49.0,FINESTEERING,2107,284049.050,02008000,471d,15824;INS_ALIGNMENT_COMPLETE,INS_RTKFIXED,37.37010717885,126.72081846735,9.9026,22.3000,-0.2042,0.1830,0.0048,-0.433320353,-1.747334753,137.205490364,0.4329,0.3030,0.5941,0.1170,0.0985,0.0797,0.0945,0.0983,5.1926,0f000001,0*334c1376\n\t", "INSPVAXA,USB3,0,49.0,FINESTEERING,2107,284049.550,02008000,471d,15824;INS_ALIGNMENT_COMPLETE,INS_RTKFIXED,37.37010620824,126.72081956922,9.9012,22.3000,-0.1970,0.1771,0.0298,-0.594531132,-1.644459886,132.097505045,0.4329,0.3030,0.5941,0.1170,0.0985,0.0797,0.0945,0.0983,5.1926,0f000001,0*6b710ba0\n\t", "INSPVAXA,USB3,0,49.0,FINESTEERING,2107,284050.050,02008000,471d,15824;INS_ALIGNMENT_COMPLETE,INS_RTKFIXED,37.37010525413,126.72082070794,9.8986,22.3000,-0.1917,0.2051,-0.0115,-0.516834592,-1.395099600,126.953212153,0.4346,0.3025,0.5938,0.1182,0.0995,0.0796,0.0941,0.0979,5.1828,0f000001,0*22942ac6\n\t", "INSPVAXA,USB3,0,50.0,FINESTEERING,2107,284050.550,02008000,471d,15824;INS_ALIGNMENT_COMPLETE,INS_RTKFIXED,37.37010440811,126.72082198518,9.8945,22.3000,-0.1594,0.2362,0.0179,-0.435131967,-1.128099811,121.559655858,0.4346,0.3025,0.5938,0.1182,0.0995,0.0796,0.0941,0.0979,5.1828,0f000001,0*78d5de76\n\t", "DUALANTENNAHEADINGA,USB3,0,50.0,FINESTEERING,2107,284051.000,02008000,d426,15824;INSUFFICIENT_OBS,NONE,-1.000000000,0.000000000,0.000000000,0.0,0.000000000,0.000000000,\"631T\",9,3,3,3,04,00,20,00*f8ed9a8f\n\t", "INSPVAXA,USB3,0,49.5,FINESTEERING,2107,284051.550,02008000,471d,15824;INS_ALIGNMENT_COMPLETE,INS_RTKFIXED,37.37010293167,126.72082506603,9.8918,22.3000,-0.2006,0.4462,0.0191,-0.487315939,-0.767469623,111.533398827,0.4366,0.3027,0.5935,0.1195,0.1007,0.0795,0.0936,0.0973,5.1774,0f000001,0*2ba22a04\n\t", "INSPVAXA,USB3,0,52.0,FINESTEERING,2107,284052.550,02000000,471d,15824;INS_ALIGNMENT_COMPLETE,INS_RTKFIXED,37.37010150239,126.72083015025,9.8922,22.3000,-0.0709,0.4201,0.0154,-1.300322363,-0.251250537,100.734835193,0.4385,0.3032,0.5931,0.1216,0.1015,0.0794,0.0930,0.0966,5.1757,0f000001,0*285f67bd\n\t", "INSPVAXA,USB3,0,51.0,FINESTEERING,2107,284053.050,02000000,471d,15824;INS_ALIGNMENT_COMPLETE,INS_RTKFIXED,37.37010109323,126.72083278272,9.8918,22.3000,-0.0521,0.4828,-0.0093,-1.553917454,-0.330463200,95.839787961,0.4397,0.3042,0.5928,0.1218,0.1030,0.0794,0.0924,0.0958,5.1723,0f000001,0*925ec3e1\n\t", "INSPVAXA,USB3,0,51.0,FINESTEERING,2107,284053.550,02000000,471d,15824;INS_ALIGNMENT_COMPLETE,INS_RTKFIXED,37.37010075654,126.72083555357,9.8892,22.3000,-0.0359,0.4357,0.0162,-0.976336983,-0.670873991,90.876153080,0.4397,0.3042,0.5928,0.1218,0.1030,0.0794,0.0924,0.0958,5.1723,0f000001,0*923600d8\n\t", "INSPVAXA,USB3,0,51.0,FINESTEERING,2107,284054.050,02000000,471d,15824;INS_ALIGNMENT_COMPLETE,INS_RTKFIXED,37.37010062155,126.72083812098,9.8896,22.3000,-0.0236,0.4683,-0.0223,-0.929923548,-0.516714504,86.855289806,0.4477,0.3075,0.5936,0.1233,0.1036,0.0794,0.0919,0.0952,5.1660,0f000001,0*98660be2\n\t", "INSPVAXA,USB3,0,52.5,FINESTEERING,2107,284054.550,02000000,471d,15824;INS_ALIGNMENT_COMPLETE,INS_RTKFIXED,37.37010072634,126.72084085451,9.8879,22.3000,0.0495,0.4621,-0.0139,-0.890595687,-0.279204622,81.540293866,0.4477,0.3075,0.5936,0.1233,0.1036,0.0794,0.0919,0.0952,5.1660,0f000001,0*57c25e6b\n\t", "INSPVAXA,USB3,0,50.5,FINESTEERING,2107,284055.050,02000000,471d,15824;INS_ALIGNMENT_COMPLETE,INS_RTKFIXED,37.37010080652,126.72084262595,9.8861,22.3000,-0.0303,0.1528,0.0096,-0.789228824,0.189504141,79.603141557,0.4534,0.3102,0.5943,0.1271,0.1038,0.0794,0.0915,0.0945,5.1589,0f000001,0*17fda88b\n\tsystem status\texception 2 27.400000 4 160\trobot status\t0.666185\t-3.261836\t9.886100\t-0.789229\t0.189504\t10.396858\t0.260000\t0.206000\n\t\n15:53:57.5\tlog_raw\tgps_raw\t#INSPVAXA,USB3,0,50.5,FINESTEERING,2107,284055.550,02000000,471d,15824;INS_ALIGNMENT_COMPLETE,INS_RTKFIXED,37.37010065353,126.72084269507,9.8843,22.3000,-0.0451,0.0165,0.0094,-0.786160418,0.167323403,79.929360762,0.4534,0.3102,0.5943,0.1271,0.1038,0.0794,0.0915,0.0945,5.1589,0f000001,0*1978198f\n\tsystem status\texception 2 27.700000 0 160\trobot status\t0.672308\t-3.278816\t9.884300\t-0.786160\t0.167323\t10.070639\t0.153000\t0.216000\n\t\n15:53:58.0\tlog_raw\tgps_raw\t#INSPVAXA,USB3,0,50.5,FINESTEERING,2107,284056.050,02000000,471d,15824;INS_ALIGNMENT_COMPLETE,INS_RTKFIXED,37.37010048956,126.72084276872,9.8836,22.3000,-0.0469,0.0143,0.0092,-0.786889601,0.175933665,79.925216666,0.4574,0.3114,0.5945,0.1322,0.1037,0.0794,0.0910,0.0937,5.1545,0f000001,0*13d22f98\n\tsystem status\texception 2 27.700000 0 160\trobot status\t0.678832\t-3.297014\t9.883600\t-0.786890\t0.175934\t10.074783\t0.147000\t0.223000\n\t\n15:53:58.5\tlog_raw\tgps_raw\t#INSPVAXA,USB3,0,51.0,FINESTEERING,2107,284056.550,02000000,471d,15824;INS_ALIGNMENT_COMPLETE,INS_RTKFIXED,37.37010037074,126.72084284514,9.8838,22.3000,-0.0480,0.0175,0.0102,-0.787820604,0.175837290,79.928422775,0.4574,0.3114,0.5945,0.1322,0.1037,0.0794,0.0910,0.0937,5.1545,0f000001,0*7f57341f\n\tsystem status\texception 2 27.700000 0 160\trobot status\t0.685601\t-3.310201\t9.883800\t-0.787821\t0.175837\t10.071577\t0.147000\t0.222000\n\t\n15:53:59.0\tlog_raw\tgps_raw\t#INSPVAXA,USB3,0,51.0,FINESTEERING,2107,284057.050,02000000,471d,15824;INS_ALIGNMENT_COMPLETE,INS_RTKFIXED,37.37010024493,126.72084294147,9.8847,22.3000,-0.0489,0.0209,0.0109,-0.790474431,0.175355820,79.934854744,0.4623,0.3124,0.5946,0.1305,0.1033,0.0793,0.0905,0.0930,5.1443,0f000001,0*1624f0ca\n\tsystem status\texception 2 27.700000 0 160\trobot status\t0.694134\t-3.324164\t9.884700\t-0.790474\t0.175356\t10.065145\t0.147000\t0.222000\n\t\n15:53:59.5\tlog_raw\tgps_raw\t#INSPVAXA,USB3,0,51.0,FINESTEERING,2107,284057.550,02000000,471d,15824;INS_ALIGNMENT_COMPLETE,INS_RTKFIXED,37.37010017546,126.72084302597,9.8865,22.3000,-0.0481,0.0245,0.0114,-0.790674154,0.175795443,79.947588667,0.4623,0.3124,0.5946,0.1305,0.1033,0.0793,0.0905,0.0930,5.1443,0f000001,0*fd60ce92\n\tsystem status\texception 2 27.700000 0 160\trobot status\t0.701619\t-3.331874\t9.886500\t-0.790674\t0.175795\t10.052411\t0.147000\t0.222000\n\t\n15:54:00.0\tlog_raw\tgps_raw\t#INSPVAXA,USB3,0,51.0,FINESTEERING,2107,284058.050,02000000,471d,15824;INS_ALIGNMENT_COMPLETE,INS_RTKFIXED,37.37010009897,126.72084313411,9.8886,22.3000,-0.0478,0.0282,0.0114,-0.793625665,0.175511830,79.961034628,0.4652,0.3130,0.5946,0.1280,0.1027,0.0793,0.0901,0.0925,5.1270,0f000001,0*11f44901\n\t", "INSPVAXA,USB3,0,52.5,FINESTEERING,2107,284058.550,02000000,471d,15824;INS_ALIGNMENT_COMPLETE,INS_RTKFIXED,37.37010007732,126.72084320054,9.8898,22.3000,-0.0461,0.0304,0.0122,-0.792445810,0.175564347,79.985489957,0.4652,0.3130,0.5946,0.1280,0.1027,0.0793,0.0901,0.0925,5.1270,0f000001,0*ea7ef511\n\tsystem status\texception 2 27.700000 0 160\trobot status\t0.717082\t-3.342766\t9.889800\t-0.792446\t0.175564\t10.014510\t0.147000\t0.222000\n\t\n15:54:01.0\tlog_raw\tgps_raw\t\tsystem status\texception 2 27.700000 0 160\trobot status\t0.724287\t-3.345631\t9.891600\t-0.792125\t0.176872\t9.990955\t0.147000\t0.222000\n\t\n15:54:01.5\tlog_raw\tgps_raw\t#INSPVAXA,USB3,0,48.0,FINESTEERING,2107,284059.550,02000000,471d,15824;INS_ALIGNMENT_COMPLETE,INS_RTKFIXED,37.37010006144,126.72084333190,9.8930,22.3000,-0.0410,0.0333,0.0137,-0.793411742,0.179299471,80.037482880,0.4658,0.3133,0.5945,0.1254,0.1019,0.0793,0.0898,0.0921,5.1054,0f000001,0*b41e64db\n\tsystem status\texception 2 27.700000 0 160\trobot status\t0.728717\t-3.344528\t9.893000\t-0.793412\t0.179299\t9.962517\t0.147000\t0.222000\n\t\n15:54:02.0\tlog_raw\tgps_raw\t#INSPVAXA,USB3,0,48.0,FINESTEERING,2107,284060.050,02000000,471d,15824;INS_ALIGNMENT_COMPLETE,INS_RTKFIXED,37.37010007091,126.72084339799,9.8948,22.3000,-0.0383,0.0348,0.0139,-0.792224776,0.181387989,80.068212083,0.4648,0.3132,0.5944,0.1230,0.1009,0.0793,0.0896,0.0921,5.0831,0f000001,0*0e446c66\n\tsystem status\texception 2 27.700000 0 160\trobot status\t0.734571\t-3.343477\t9.894800\t-0.792225\t0.181388\t9.931788\t0.147000\t0.222000\n\t\n15:54:02.5\tlog_raw\tgps_raw\t#INSPVAXA,USB3,0,51.5,FINESTEERING,2107,284060.550,02000000,471d,15824;INS_ALIGNMENT_COMPLETE,INS_RTKFIXED,37.37010010371,126.72084343010,9.8965,22.3000,-0.0351,0.0351,0.0141,-0.794008331,0.181387588,80.099175193,0.4648,0.3132,0.5944,0.1230,0.1009,0.0793,0.0896,0.0921,5.0831,0f000001,0*6d5ef346\n\tsystem status\texception 2 27.700000 0 160\trobot status\t0.737416\t-3.339837\t9.896500\t-0.794008\t0.181388\t9.900825\t0.147000\t0.222000\n\t\n15:54:03.0\tlog_raw\tgps_raw\t#INSPVAXA,USB3,0,47.0,FINESTEERING,2107,284061.050,02000000,471d,15824;INS_ALIGNMENT_COMPLETE,INS_RTKFIXED,37.37010013657,126.72084347859,9.8982,22.3000,-0.0318,0.0362,0.0140,-0.793134778,0.182296813,80.130371651,0.4625,0.3128,0.5942,0.1207,0.0997,0.0793,0.0895,0.0922,5.0625,0f000001,0*150e9f64\n\tsystem status\texception 2 27.700000 0 160\trobot status\t0.741711\t-3.336190\t9.898200\t-0.793135\t0.182297\t9.869628\t0.147000\t0.222000\n\t\n15:54:03.5\tlog_raw\tgps_raw\t\tsystem status\texception 2 27.700000 0 160\trobot status\t0.745103\t-3.333746\t9.898900\t-0.794686\t0.183659\t9.841140\t0.147000\t0.222000\n\t\n15:54:04.0\tlog_raw\tgps_raw\t#INSPVAXA,USB3,0,47.0,FINESTEERING,2107,284062.050,02000000,471d,15824;INS_ALIGNMENT_COMPLETE,INS_RTKFIXED,37.37010017748,126.72084356719,9.8997,22.3000,-0.0290,0.0363,0.0139,-0.794331592,0.183823168,80.187481896,0.4594,0.3121,0.5941,0.1189,0.0986,0.0793,0.0895,0.0925,5.0451,0f000001,0*0cfca1c0\n\tsystem status\texception 2 27.800000 0 160\trobot status\t0.749559\t-3.331650\t9.899700\t-0.794332\t0.183823\t9.812518\t0.147000\t0.222000\n\t\n15:54:04.5\tlog_raw\tgps_raw\t\tsystem status\texception 2 27.700000 0 160\trobot status\t0.750935\t-3.327984\t9.900000\t-0.792965\t0.186753\t9.783400\t0.147000\t0.222000\n\t\n15:54:05.0\tlog_raw\tgps_raw\t#INSPVAXA,USB3,0,47.5,FINESTEERING,2107,284063.050,02000000,471d,15824;INS_ALIGNMENT_COMPLETE,INS_RTKFIXED,37.37010026095,126.72084358162,9.8989,22.3000,-0.0250,0.0360,0.0144,-0.793980547,0.188879000,80.251853132,0.3252,0.2278,0.4744,0.0459,0.0444,0.0422,0.0723,0.0737,4.9906,0f000005,0*164f8940\n\t", "INSPVAXA,USB3,0,47.5,FINESTEERING,2107,284063.550,02000000,471d,15824;INS_ALIGNMENT_COMPLETE,INS_RTKFIXED,37.37010060191,126.72084312304,9.8728,22.3000,-0.0145,0.0225,0.0107,-0.798483661,0.197892830,80.372723663,0.3252,0.2278,0.4744,0.0459,0.0444,0.0422,0.0723,0.0737,4.9906,0f000005,0*92bf4382\n\tsystem status\texception 2 27.700000 0 160\trobot status\t0.710217\t-3.284545\t9.872800\t-0.798484\t0.197893\t9.627276\t0.147000\t0.222000\n\t\n15:54:06.0\tlog_raw\tgps_raw\t#INSPVAXA,USB3,0,47.5,FINESTEERING,2107,284064.050,02000000,471d,15824;INS_ALIGNMENT_COMPLETE,INS_RTKFIXED,37.37010092341,126.72084268927,9.8479,22.3000,-0.0050,0.0083,0.0065,-0.802010918,0.203072267,80.489552578,0.3043,0.2119,0.4435,0.0375,0.0370,0.0348,0.0717,0.0735,4.9827,0f000005,0*2a9229fa\n\tsystem status\texception 2 27.700000 0 160\trobot status\t0.671794\t-3.248863\t9.847900\t-0.802011\t0.203072\t9.510447\t0.147000\t0.222000\n\t\n15:54:06.5\tlog_raw\tgps_raw\t#INSPVAXA,USB3,0,52.0,FINESTEERING,2107,284064.550,02000000,471d,15824;INS_ALIGNMENT_COMPLETE,INS_RTKFIXED,37.37010093886,126.72084266042,9.8416,22.3000,-0.0043,0.0064,0.0059,-0.803970150,0.202555305,80.508100729,0.3043,0.2119,0.4435,0.0375,0.0370,0.0348,0.0717,0.0735,4.9827,0f000005,0*b303c02a\n\tsystem status\texception 2 27.800000 0 160\trobot status\t0.669239\t-3.247148\t9.841600\t-0.803970\t0.202555\t9.491899\t0.147000\t0.222000\n\t\n15:54:07.0\tlog_raw\tgps_raw\t#INSPVAXA,USB3,0,48.0,FINESTEERING,2107,284065.050,02000000,471d,15824;INS_ALIGNMENT_COMPLETE,INS_RTKFIXED,37.37010095172,126.72084263427,9.8359,22.3000,-0.0031,0.0050,0.0058,-0.803101201,0.203067002,80.525514277,0.2907,0.2017,0.4242,0.0352,0.0350,0.0325,0.0719,0.0737,4.9778,0f000005,0*fc85e648\n\t", "INSPVAXA,USB3,0,50.0,FINESTEERING,2107,284066.550,02000000,471d,15824;INS_ALIGNMENT_COMPLETE,INS_RTKFIXED,37.37010094761,
